vi "DHE_Stop.vi"(6 "DHE_DBSRef":T1, 8 "error in (no error)":errorcluster, 10 "args":string, 11 "fd":i32) -> (0 "error out":errorcluster, 2 "return value":i32, 3 "fd out":i32)   [LabVIEW 2016]
uses:
  DBSHAND/private/vis/DatabaseHand_RefNum.ctl
  DBSHAND/private/vis/DatabaseHand_Element_Get(bool).vi
panel:
  in  "phys unit":string
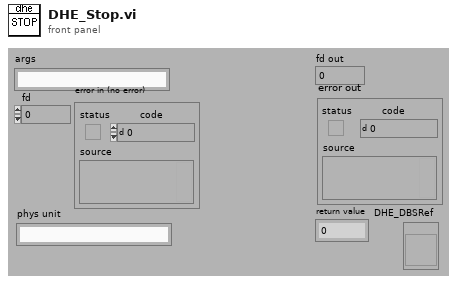
[diagram p1: front panel]
types:
  T1 = typedef "DatabaseHand_RefNum.ctl" = refnum<vi>
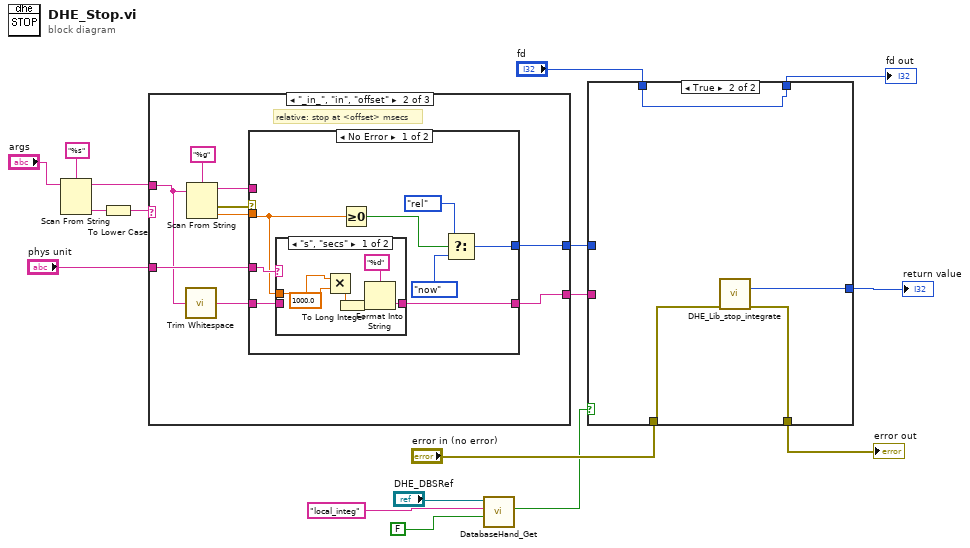
[diagram p0: block diagram]
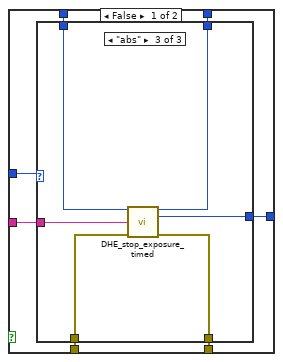
[diagram p2: hidden frame]
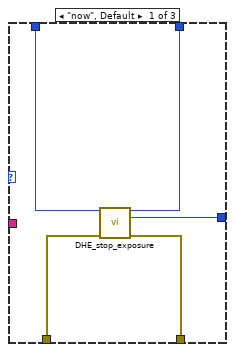
[diagram p3: hidden frame]
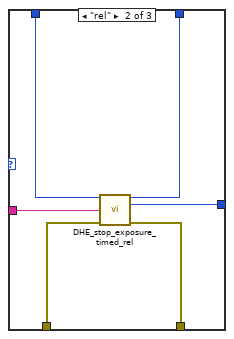
[diagram p4: hidden frame]
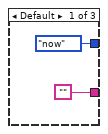
[diagram p5: hidden frame]
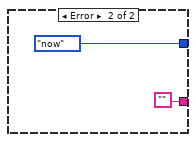
[diagram p7: hidden frame]
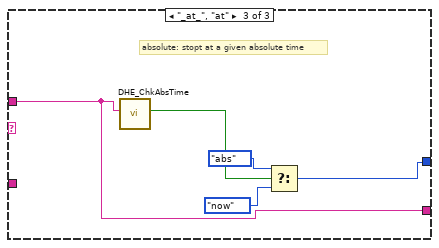
[diagram p8: hidden frame]
diagram:
  n1 = Scan From String(format string="%s", input string="args") -> (remaining string=w13:string, output 1=w15:string)  [unwired: 2 in, 3 out]
  n2 = To Lower Case(string=w15) -> (all lower case string=w14:string)
  n3 = case shown="\"_in_\", \"in\", \"offset\"" w14 {
    tunnel: w13 -> [_ w22 w47]
    tunnel: [enum16{"now", "abs", "rel"}."now" w26 w48] -> w12
    tunnel: ["" w21 w47] -> w6
    tunnel: "phys unit" -> [_ w23 _]
    frame Default {
    }
    frame "_in_", "in", "offset" {
      # "relative: stop at <offset> msecs"
      n4 = call <vilib>:"Trim Whitespace.vi"("string"=w22) -> ("trimmed string"=w20:string)  [unwired: 1 in]
      n5 = Scan From String(format string="%g", input string=w22) -> (remaining string=w24:string, error out=w27:errorcluster, output 1=w25:dbl)  [unwired: 2 in, 2 out]
      n6 = case shown="No Error" w27 {
        tunnel: [w33 enum16{"now", "abs", "rel"}."now"] -> w26
        tunnel: w25 -> [w31 _]
        tunnel: w24 -> [_ _]
        tunnel: w23 -> [w32 _]
        tunnel: w20 -> [w30 _]
        tunnel: [w29 ""] -> w21
        frame No Error {
          n7 = case shown="\"s\", \"secs\"" w32 {
            tunnel: w31 -> [w42 _]
            tunnel: w30 -> [_ w43]
            tunnel: [w39 w43] -> w29
            frame "s", "secs" {
              n8 = Multiply(x=w42, y=1000.0) -> (x*y=w40:dbl)
              n9 = To Long Integer(number=w40) -> (32bit integer=w37:i32)
              n10 = Format Into String(format string="%d", w37) -> (resulting string=w39:string)  [unwired: 2 in, 1 out]
            }
            frame "", Default {
            }
          }
          n11 = Greater Or Equal To 0?(x=w31) -> (x >= 0?=w36:bool)
          n12 = Select(t=enum16{"now", "abs", "rel"}."rel", s=w36, f=enum16{"now", "abs", "rel"}."now") -> (s? t:f=w33:enum16{"now", "abs", "rel"})
        }
        frame Error {
        }
      }
    }
    frame "_at_", "at" {
      # "absolute: stopt at a given absolute time"
      n13 = call "DHE_ChkAbsTime.vi"("abstime"=w47) -> ("ok"=w50:bool)  [unwired: 10 out]
      n14 = Select(t=enum16{"now", "abs", "rel"}."abs", s=w50, f=enum16{"now", "abs", "rel"}."now") -> (s? t:f=w48:enum16{"now", "abs", "rel"})
    }
  }
  n15 = call-poly "DatabaseHand_Get.vi"("default value"=FALSE, "name"="local_integ", "Database RefNum in"="DHE_DBSRef") -> ("value"=w1:bool)  [unwired: 2 in, 6 out]
  n16 = case shown="True" w1 {
    tunnel: w12 -> [w57 _]
    tunnel: "error in (no error)" -> [w56 w77]
    tunnel: [w55 w76] -> w10
    tunnel: "fd" -> [w54 w78]
    tunnel: [w53 w78] -> w8
    tunnel: [w52 w75] -> w7
    tunnel: w6 -> [w51 _]
    frame False {
      n17 = case shown="\"abs\"" w57 {
        tunnel: w56 -> [w62 w68 w74]
        tunnel: [w61 w67 w73] -> w55
        tunnel: w54 -> [w60 w66 w72]
        tunnel: [w59 w65 w71] -> w53
        tunnel: [w58 w64 w70] -> w52
        tunnel: w51 -> [_ w63 w69]
        frame "now", Default {
          n18 = call "DHE_stop_exposure.vi"("fd"=w60, "error in (no error)"=w62) -> ("fd out"=w59:i32, "return value"=w58:i32, "error out"=w61:errorcluster)  [unwired: 1 in, 10 out]
        }
        frame "rel" {
          n19 = call "DHE_stop_exposure_timed_rel.vi"("fd"=w66, "offset(msecs)"=w63, "error in (no error)"=w68) -> ("fd out"=w65:i32, "return value"=w64:i32, "error out"=w67:errorcluster)  [unwired: 10 out]
        }
        frame "abs" {
          n20 = call "DHE_stop_exposure_timed.vi"("fd"=w72, "stop_time"=w69, "error in (no error)"=w74) -> ("fd out"=w71:i32, "return value"=w70:i32, "error out"=w73:errorcluster)  [unwired: 10 out]
        }
      }
    }
    frame True {
      n21 = call "DHE_Lib_stop_integrate.vi"("error in (no error)"=w77) -> ("actual integ"=w75:i32, "error out"=w76:errorcluster)  [unwired: 13 out]
    }
  }
  "fd out" <- w8
  "error out" <- w10
  "return value" <- w7
